vi "read multiple params.vi"(8 "error in (no error)":errorcluster, 10 "Parameters":u32[](array[numeric]) format="%.0x", 11 "Stepper in":refnum<class "Stepper.lvclass">) -> (0 "error out":errorcluster, 2 "Hex Result":u32[](array[numeric]) format="%.0x", 3 "Stepper out":refnum<class "Stepper.lvclass">)   [LabVIEW 2025, in "Stepper.lvclass"]
uses:
  Stepper.lvclass
  Stepper.lvclass/Stepper.ctl
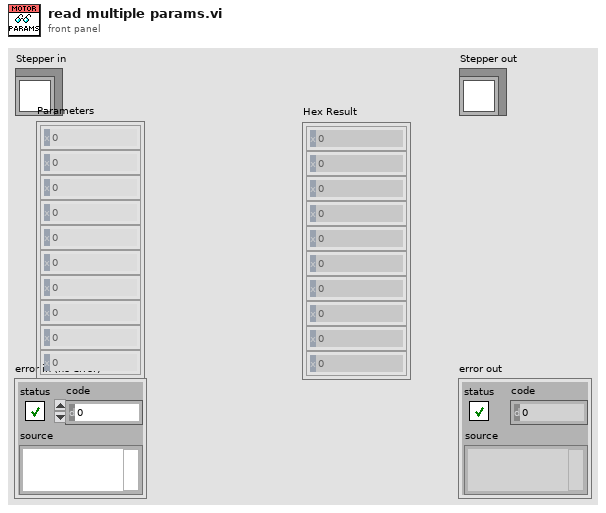
[diagram p1: front panel]
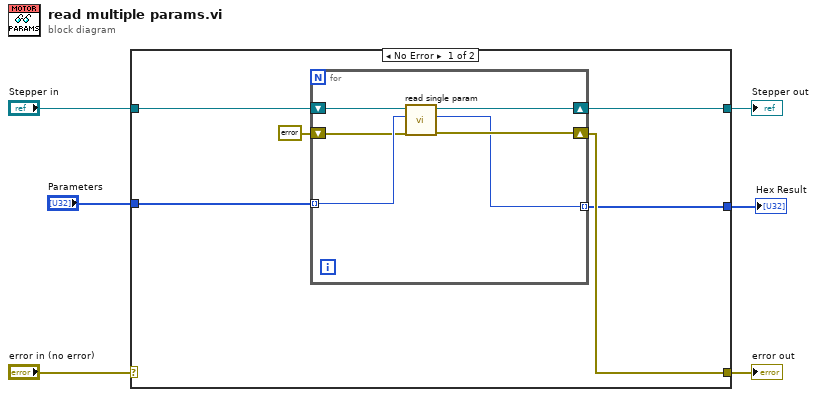
[diagram p0: block diagram]
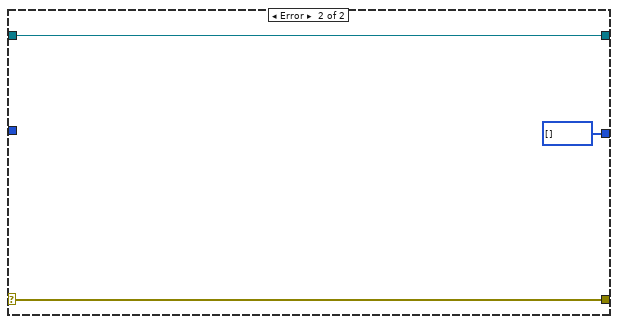
[diagram p2: hidden frame]
diagram:
  n1 = case shown="No Error" "error in (no error)" {
    selector: "error in (no error)" -> [_ w21]
    tunnel: [w10 w21] -> w5
    tunnel: [w9 w20] -> w3
    tunnel: "Stepper in" -> [w11 w20]
    tunnel: "Parameters" -> [w12 _]
    tunnel: [w8 u16[] []] -> w1
    frame No Error {
      n2 = for {
        tunnel: w12 -> [w17] mode=indexing
        shift-right: [w15] -> w10
        shift-left: errorcluster {"status"=FALSE, "code"=0, "source"=""} ("error out") -> [w16]
        shift-right: [w14] -> w9
        shift-left: w11 -> [w18]
        tunnel: [w13] -> w8 mode=indexing
        n3 = call-dynamic "read single param.vi"("error in (no error)"=w16, "address"=w17, "Stepper in"=w18) -> ("error out"=w15:errorcluster, "register"=w13:u16, "Stepper out"=w14:refnum<class "Stepper.lvclass">)  [unwired: 6 in]
      }
    }
    frame Error {
    }
  }
  "error out" <- w5
  "Stepper out" <- w3
  "Hex Result" <- w1
